vi "Base Tree Tests.vi"(8 "error in (no error)":errorcluster) -> (0 "error out":errorcluster)   [LabVIEW 2017, in "Unit Tests.lvlib"]
uses:
  Unit Tests.lvlib
  <vilib>/addons/_JKI Toolkits/Caraya/classes/Test/Test.lvclass
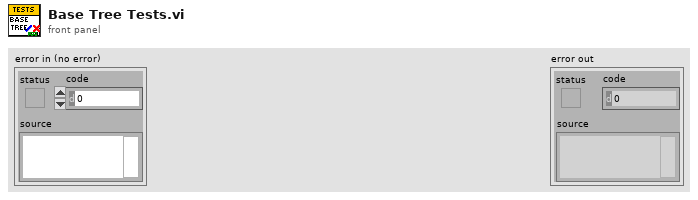
[diagram p1: front panel]
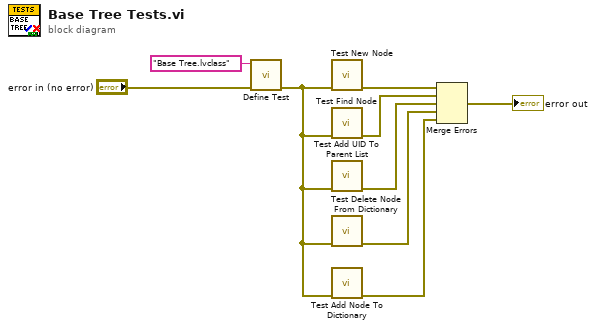
[diagram p0: block diagram]
diagram:
  n1 = call <vilib>:"Define Test.vi"("error in (no error)"="error in (no error)", "Label (VI Title)"="Base Tree.lvclass") -> ("error out"=w2:errorcluster)  [unwired: 9 in]
  n2 = call "Test New Node.vi"("error in (no error)"=w2) -> ("error out"=w7:errorcluster)  [unwired: 10 in]
  n3 = call "Test Find Node.vi"("error in (no error)"=w2) -> ("error out"=w5:errorcluster)  [unwired: 10 in]
  n4 = call "Test Add UID To Parent List.vi"("error in (no error)"=w2) -> ("error out"=w4:errorcluster)  [unwired: 10 in]
  n5 = call "Test Delete Node From Dictionary.vi"("error in (no error)"=w2) -> ("error out"=w3:errorcluster)  [unwired: 10 in]
  n6 = call "Test Add Node To Dictionary.vi"("error in (no error)"=w2) -> ("error out"=w1:errorcluster)  [unwired: 10 in]
  n7 = Merge Errors(w7, w5, w4, w3, w1) -> (→"error out":errorcluster)
